vi "Finish Update.vi"(8 "instVIref":T1, 11 "RTTarget in":refnum<class "RTTarget.lvclass">) -> (3 "RTTarget out":refnum<class "RTTarget.lvclass">)   [LabVIEW 2020, in "NI_TargetHelper.lvlib" / "RTTarget.lvclass"]
uses:
  <vilib>/TargetSupport/NI_TargetHelper/RTTarget/RTTarget.lvclass
  <vilib>/TargetSupport/NI_TargetHelper/Instance VIref.ctl
  <vilib>/Utility/miscctls.llb/LVPointTypeDef.ctl
  <vilib>/TargetSupport/NI_TargetHelper/RTTarget/RTTarget.lvclass/RTTarget.ctl
  <vilib>/TargetSupport/NI_TargetHelper/NI_TargetHelper.lvlib
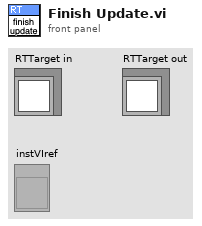
[diagram p1: front panel]
types:
  T1 = typedef "NI_TargetHelper.lvlib/Instance VIref.ctl" = refnum<vi>
  T2 = typedef "LVPointTypeDef.ctl" = cluster{"Horizontal":i16, "Vertical":i16}
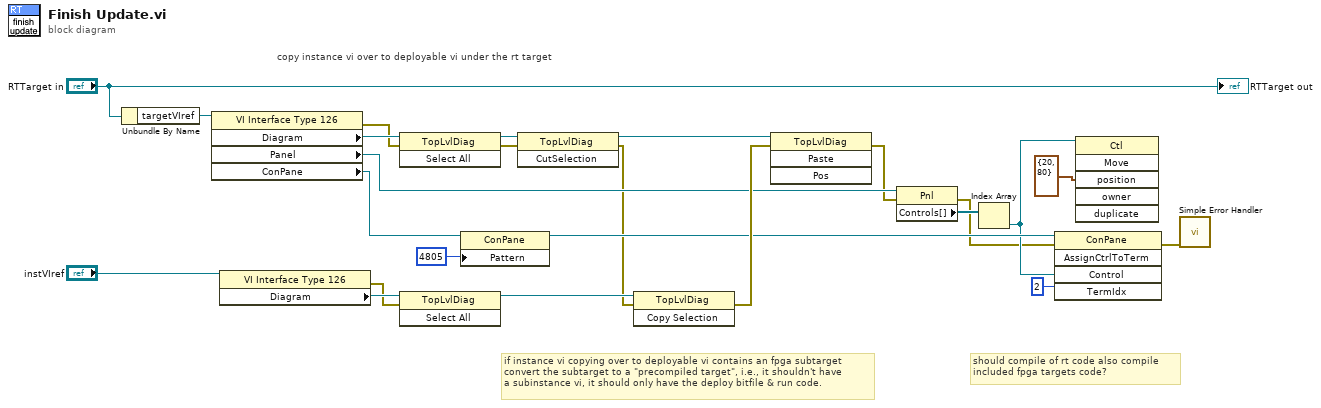
[diagram p0: block diagram]
diagram:
  # "should compile of rt code also compile\nincluded fpga targets code?"
  # "if instance vi copying over to deployable vi contains an fpga subtarget\nconvert the subtarget to a \"precompiled target\", i.e., it shouldn't have \na subinstance vi, it should only have the deploy bitfile & run code."
  # "copy instance vi over to deployable vi under the rt target"
  n1 = Unbundle By Name("RTTarget in") -> ("targetVIref"=w23:T1)
  n2 = property class="VI Interface Type 126"(reference=w23) -> (error out=w5:errorcluster, "Diagram"=w22:refnum<vi>, "Panel"=w12:refnum<vi>, "ConPane"=w15:refnum<vi>)  [unwired: 1 in, 1 out]
  n3 = property class="VI Interface Type 126"(reference="instVIref") -> (error out=w6:errorcluster, "Diagram"=w19:refnum<vi>)  [unwired: 1 in, 1 out]
  n4 = invoke class="TopLvlDiag" method="Select All"(reference=w22, error in=w5) -> (reference out=w21:refnum<vi>, error out=w4:errorcluster)  [unwired: 1 in, 1 out]
  n5 = invoke class="TopLvlDiag" method="Select All"(reference=w19, error in=w6) -> (reference out=w20:refnum<vi>)  [unwired: 1 in, 2 out]
  n6 = property class="ConPane"(reference=w15, "Pattern"=u32 4805) -> (reference out=w13:refnum<vi>)  [unwired: 1 in, 1 out]
  n7 = invoke class="TopLvlDiag" method="CutSelection"(reference=w21, error in=w4) -> (reference out=w18:refnum<vi>, error out=w1:errorcluster)  [unwired: 1 in, 1 out]
  n8 = invoke class="TopLvlDiag" method="Copy Selection"(reference=w20, error in=w1) -> (error out=w17:errorcluster)  [unwired: 1 in, 2 out]
  n9 = invoke class="TopLvlDiag" method="Paste"(reference=w18, error in=w17) -> (error out=w10:errorcluster)  [unwired: 2 in, 3 out]
  n10 = property class="Pnl"(reference=w12, error in=w10) -> (error out=w3:errorcluster, "Controls[]"=w11:refnum<vi>[])  [unwired: 1 out]
  n11 = Index Array(array=w11) -> (element=w8:refnum<vi>)  [unwired: 1 in]
  n12 = invoke class="ConPane" method="AssignCtrlToTerm"(reference=w13, error in=w3, "Control"=w8, "TermIdx"=u32 2 ("Terminal Index")) -> (error out=w2:errorcluster)  [unwired: 1 in, 4 out]
  n13 = invoke class="Ctl" method="Move"(reference=w8, "position"=T2 {"Horizontal"=20, "Vertical"=80} ("location")) -> ()  [unwired: 4 in, 6 out]
  n14 = call <vilib>:"Simple Error Handler.vi"("error in (no error)"=w2) -> ()  [unwired: 4 in, 5 out]
  "RTTarget out" <- "RTTarget in"
